vi "Do.vi"(8 "error in (no error)":errorcluster, 10 "Actor in":refnum<class "Actor.lvclass">, 11 "Receive Response Msg":refnum<class "Receive Response Msg.lvclass">) -> (0 "error out":errorcluster, 2 "Actor out":refnum<class "Actor.lvclass">)   [LabVIEW 2019, in "Power Supply.lvlib" / "Receive Response Msg.lvclass"]
doc: "This VI delivers the message to the actor by calling the appropriate method(s) on the actor."
uses:
  Receive Response Msg.lvclass
  C:/Working Copy/trunk/Modified Cobra Jung/Cobra/Cobra AF/Serial/Serial Messages/Response Msg/Response Msg.lvclass
  <vilib>/ActorFramework/Actor/Actor.lvclass
  Power Supply/Power Supply.lvclass
  C:/Program Files (x86)/National Instruments/LabVIEW 2019/vi.lib/ActorFramework/Actor/Actor.lvclass
  Serial/Serial Messages/Response Msg/Response Msg.lvclass/Response Msg.ctl
  Serial/Serial Messages/Response Msg/Response Msg.lvclass
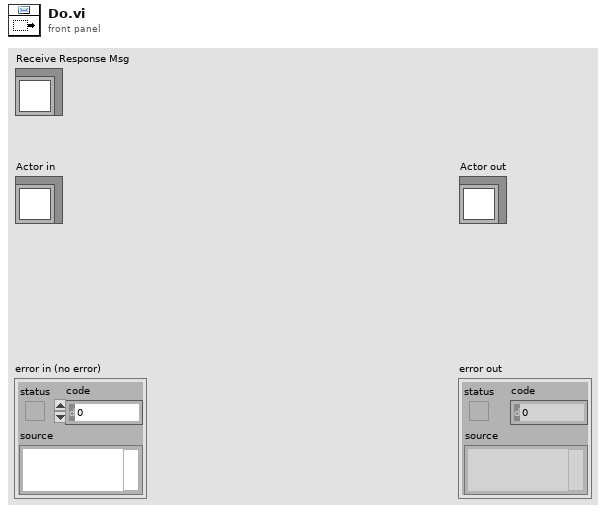
[diagram p1: front panel]
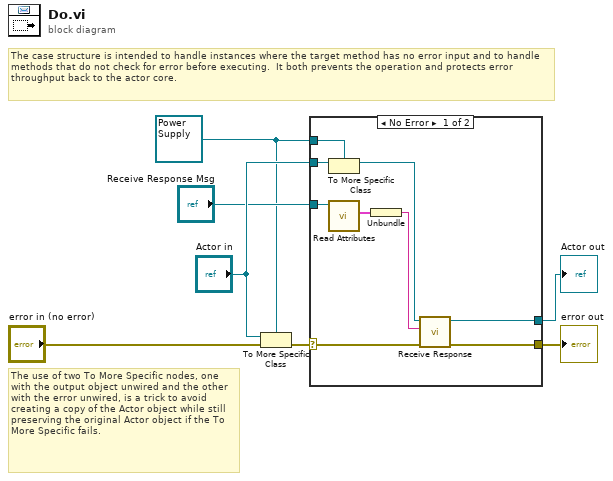
[diagram p0: block diagram]
diagram:
  w1 = refnum<class "Power Supply.lvclass"> refnum ("Power Supply.lvlib:Power Supply.lvclass")
  # "The use of two To More Specific nodes, one with the output object unwired and the other with the error unwired, is a trick to avoid creating a copy of the Actor object while still preserving the original Actor object if the To More Specific fails."
  # "The case structure is intended to handle instances where the target method has no error input and to handle methods that do not check for error before executing.  It both prevents the operation and protects error throughput back to the actor core."
  n1 = To More Specific Class(target class=w1, reference="Actor in", error in="error in (no error)") -> (error out=w6:errorcluster)  [unwired: 1 out]
  n2 = case shown="No Error" w6 {
    selector: w6 -> [w14 w18]
    tunnel: [w16 w18] -> w5
    tunnel: [w15 w17] -> w4
    tunnel: "Actor in" -> [w13 w17]
    tunnel: w1 -> [w12 _]
    tunnel: "Receive Response Msg" -> [w9 _]
    frame No Error {
      n3 = To More Specific Class(target class=w12, reference=w13) -> (specific class reference=w11:refnum<class "Power Supply.lvclass">)  [unwired: 1 in, 1 out]
      n4 = call "Read Attributes.vi"("Response Msg"=w9) -> ("Payload"=w10:cluster{"Response":string})  [unwired: 10 in]
      n5 = Unbundle(w10) -> ("Response"=w8:string)
      n6 = call "Receive Response.vi"("error in"=w14, "Response"=w8, "PS in"=w11) -> ("error out"=w16:errorcluster, "PS out"=w15:refnum<class "Power Supply.lvclass">)  [unwired: 7 in]
    }
    frame Error {
      # "If type check fails, pass the original object out again."
    }
  }
  "error out" <- w5
  "Actor out" <- w4
